vi "AlGaInPAs_Layer_v01.vi"(0 "Al run":bool, 1 "Al Flow":dbl, 2 "In run":bool, 3 "Ga run":bool, 4 "Ga Flow":dbl, 5 "PH3 run":bool, 6 "PH3 Flow":dbl, 7 "In Flow":dbl, 8 "AsH3 run":bool, 9 "AsH3 Flow":dbl) -> ()   [LabVIEW 2011]
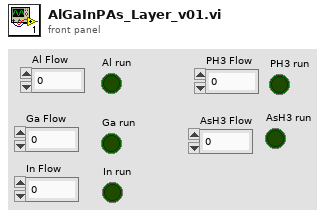
[diagram p1: front panel]
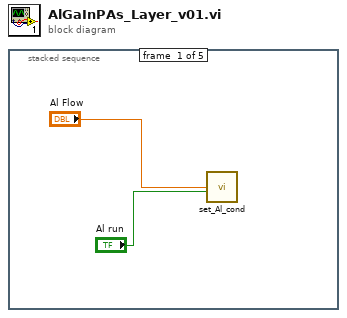
[diagram p0: block diagram]
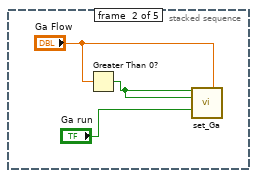
[diagram p2: hidden frame]
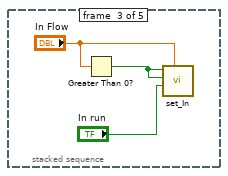
[diagram p3: hidden frame]
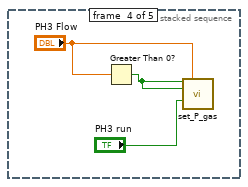
[diagram p4: hidden frame]
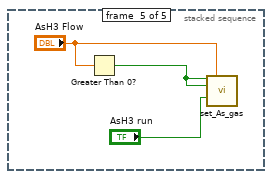
[diagram p5: hidden frame]
diagram:
  n1 = stacked-sequence {
    frame #0 {
      n2 = call "set_Al_cond.vi"("Aluminum Flow"="Al Flow", "Al Run"="Al run") -> ()  [unwired: 8 in]
    }
    frame #1 {
      n3 = Greater Than 0?(x="Ga Flow") -> (x > 0?=w3:bool)
      n4 = call "set_Ga.vi"("Ga Active"=w3, "Ga Flow 1"="Ga Flow", "Ga Bubbler"=w3, "Ga Run"="Ga run") -> ()  [unwired: 4 in, 8 out]
    }
    frame #2 {
      n5 = Greater Than 0?(x="In Flow") -> (x > 0?=w6:bool)
      n6 = call "set_In.vi"("Indium Flow"="In Flow", "In Run"="In run", "In Bubbler"=w6, "In Active"=w6) -> ()  [unwired: 1 in, 5 out]
    }
    frame #3 {
      n7 = Greater Than 0?(x="PH3 Flow") -> (x > 0?=w9:bool)
      n8 = call "set_P_gas.vi"("P_Gas Active"=w9, "P_Gas Flow"="PH3 Flow", "P_Gas In"=w9, "P_Gas Run"="PH3 run") -> ()  [unwired: 2 in, 10 out]
    }
    frame #4 {
      n9 = Greater Than 0?(x="AsH3 Flow") -> (x > 0?=w12:bool)
      n10 = call "set_As_gas.vi"("As_Gas Active"=w12, "As_Gas Flow"="AsH3 Flow", "As_Gas In"=w12, "As_Gas Run"="AsH3 run") -> ()  [unwired: 2 in, 10 out]
    }
  }
